vi "RLC_read_C_S1_2.vi"() -> (0 "MEASURE C [F ]":dbl, 1 "MEASURE V [V]":dbl, 2 "concatenated string":string, 3 "READ RLC300 - digimess":string, 4 "MEASURE R [Ohm ]":dbl, 5 "MEASURE I [A]":dbl)   [LabVIEW 2011]
panel:
  out "EXPOENTE I":dbl
  out "VALOR I":dbl
  out "EXPOENTE V":dbl
  out "VALOR V":dbl
  out "EXPOENTE R":dbl
  out "VALOR R":dbl
  out "EXPOENTE C":dbl
  out "VALOR C":dbl
  out "SEGUNDO":dbl
  out "MINUTO":dbl
  out "HORA":dbl
  out "ANO":dbl
  out "DIA":dbl
  out "MES":dbl
  out "Output Strings":string[](array[string])
  out "Output Numbers":dbl[](array[numeric]) format="%0.2f"
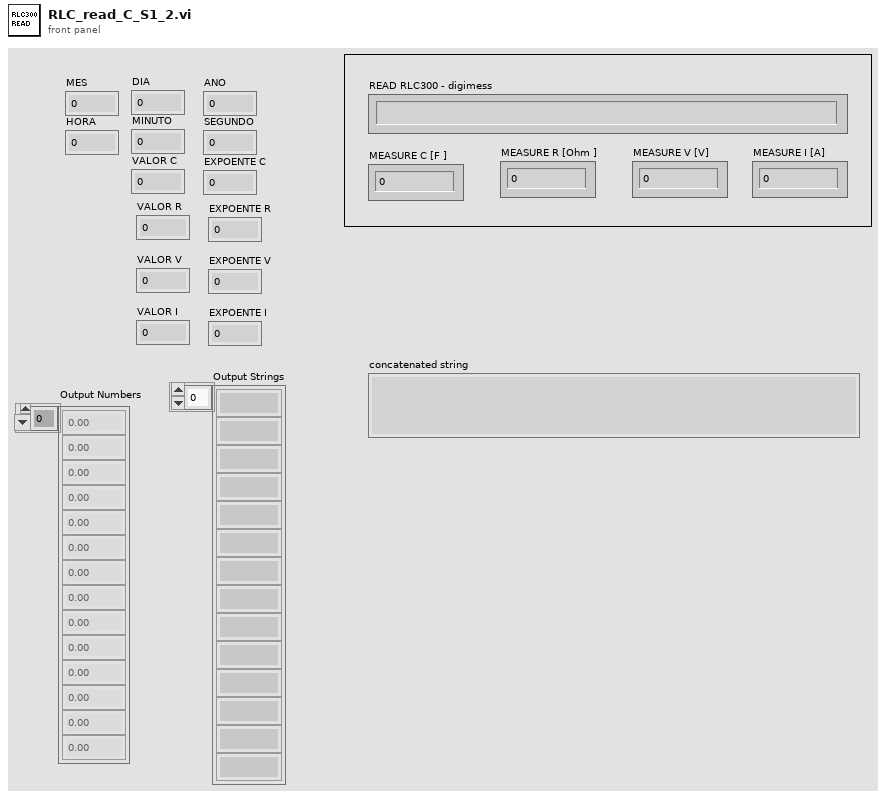
[diagram p1: front panel]
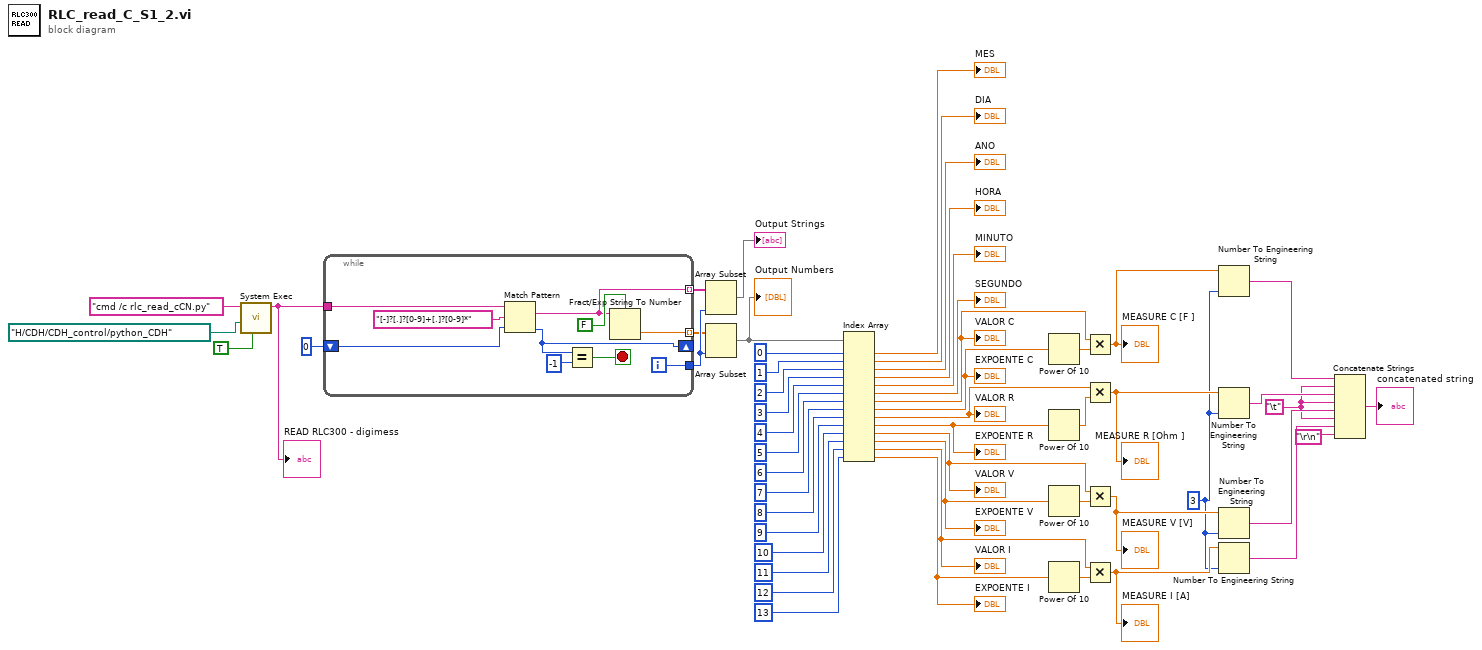
[diagram p0: block diagram]
diagram:
  w1 = i16 3 ("precision (6)")
  w5 = "\t"
  n1 = call <vilib>:"System Exec.vi"("run minimized? (F)"=TRUE, "working directory"=path "H:/CDH/CDH_control/python_CDH" ("Path"), "command line"="cmd /c rlc_read_cCN.py") -> ("standard output"=w28:string)  [unwired: 5 in, 3 out]
  "READ RLC300 - digimess" <- w28
  n2 = while {
    tunnel: [w64] -> w39
    shift-left: 0 -> [w59]
    shift-right: [w58] -> _
    tunnel: [w62] -> w38 mode=indexing
    tunnel: [w56] -> w40 mode=indexing
    tunnel: w28 -> [w55]
    i -> [w64]
    stop <- w61 stop-if-true
    n3 = Match Pattern(string=w55, regular expression="[-]?[.]?[0-9]+[.]?[0-9]*", offset (0)=w59) -> (match substring=w56:string, offset past match=w58:i32)  [unwired: 2 out]
    n4 = Equal?(x=w58, y=-1) -> (x = y?=w61:bool)
    n5 = Fract/Exp String To Number(use system decimal point (T)=FALSE, string=w56) -> (number=w62:dbl)  [unwired: 2 in, 1 out]
  }
  n6 = Array Subset(array=w40, length=w39) -> (→"Output Strings":string[])  [unwired: 1 in]
  n7 = Array Subset(array=w38, length=w39) -> (w43:dbl[])  [unwired: 1 in]
  "Output Numbers" <- w43
  n8 = Index Array(array=w43, index #1=0, index #2=1, index #3=2, index #4=3, index #5=4, index #6=5, index #7=6, index #8=7, index #9=8 ("index"), index #10=9 ("index"), index #11=10 ("index"), index #12=11 ("index"), index #13=12 ("index"), index #14=13 ("index")) -> (element #1=→"MES":dbl, element #2=→"DIA":dbl, element #3=→"ANO":dbl, element #4=→"HORA":dbl, element #5=→"MINUTO":dbl, element #6=→"SEGUNDO":dbl, element #7=w29:dbl, element #8=w30:dbl, element #9=w24:dbl, element #10=w23:dbl, element #11=w19:dbl, element #12=w18:dbl, element #13=w14:dbl, element #14=w13:dbl)
  "VALOR C" <- w29
  "EXPOENTE C" <- w30
  "VALOR R" <- w24
  "EXPOENTE R" <- w23
  "VALOR V" <- w19
  "EXPOENTE V" <- w18
  "VALOR I" <- w14
  "EXPOENTE I" <- w13
  n9 = Power Of 10(x=w30) -> (10^x=w51:dbl)
  n10 = Power Of 10(x=w23) -> (10^x=w25:dbl)
  n11 = Power Of 10(x=w18) -> (10^x=w22:dbl)
  n12 = Power Of 10(x=w13) -> (10^x=w17:dbl)
  n13 = Multiply(x=w29, y=w51) -> (x*y=w12:dbl)
  "MEASURE C [F ]" <- w12
  n14 = Multiply(x=w24, y=w25) -> (x*y=w9:dbl)
  "MEASURE R [Ohm ]" <- w9
  n15 = Multiply(x=w19, y=w22) -> (x*y=w10:dbl)
  "MEASURE V [V]" <- w10
  n16 = Multiply(x=w14, y=w17) -> (x*y=w11:dbl)
  "MEASURE I [A]" <- w11
  n17 = Number To Engineering String(2:w1, 4:w12) -> (0:w8:string)  [unwired: 2 in]
  n18 = Number To Engineering String(2:w1, 4:w9) -> (0:w7:string)  [unwired: 2 in]
  n19 = Number To Engineering String(2:w1, 4:w10) -> (0:w6:string)  [unwired: 2 in]
  n20 = Number To Engineering String(2:w1, 4:w11) -> (0:w4:string)  [unwired: 2 in]
  n21 = Concatenate Strings(w8, w5, w7, w5, w6, w5, w4, "\r\n") -> (→"concatenated string":string)
